vi "WM Spectra Stroke Calibration.vi"(0 "Input Time Series":dbl[](array[numeric]) format="%.2f", 1 "Water Depth":dbl format="%.2f", 2 "Sampling Rate":dbl format="%.2f", 3 "Paddle Height":dbl format="%.2f", 4 "Conversion Type":u16(ring) items=["Wave Height to Stroke", "Stroke to Wave Height"]) -> (5 "Output Time Series":dbl[](array[numeric]) format="%.2f")   [LabVIEW 2012]
uses:
  <vilib>/Analysis/2dsp.llb/Real FFT.vi
  <vilib>/Analysis/2dsp.llb/Inverse Real FFT.vi
  <vilib>/Analysis/NI_AALPro.lvlib
panel:
  # "Flap Stroke at Water line (S)"
  # "Flap Amplitude From x=0 (A')"
  # "Total Flap Stroke (S')"
  # "Flap Height (h')"
  # "Wave Height (Peak to trough) (H)"
  # "Wave Amplitude (z=0 to Peak) (A)"
  # "Wave Height to Flap Stroke at Water Line ( [H/S] )"
  # "Water Depth (h)"
  # "A' = h' * H / ( 2 * h * [H/S] )"
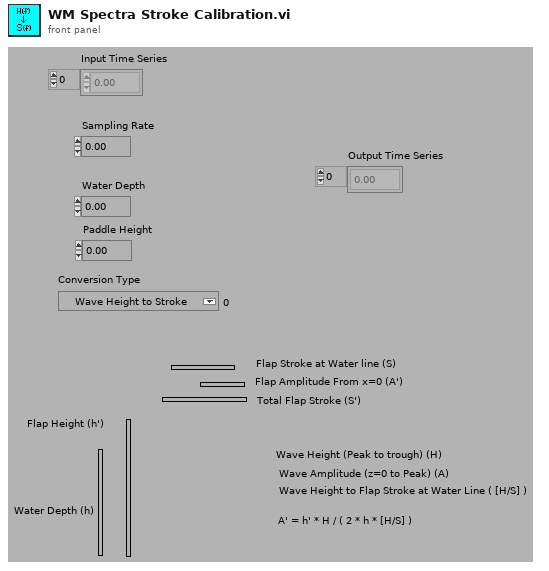
[diagram p1: front panel]
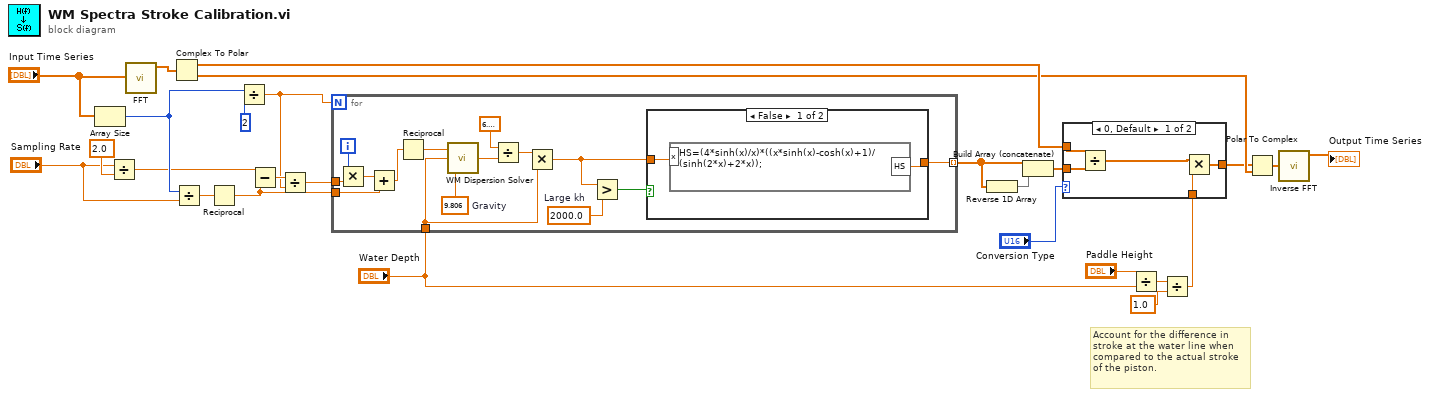
[diagram p0: block diagram]
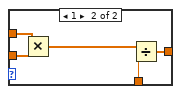
[diagram p2: hidden frame]
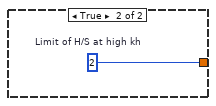
[diagram p3: hidden frame]
diagram:
  # "Account for the difference in \nstroke at the water line when \ncompared to the actual stroke\nof the piston."
  n1 = Array Size(array="Input Time Series") -> (size(s)=w14:i32)
  n2 = Divide(x="Sampling Rate", y=2.0) -> (x/y=w13:dbl)
  n3 = call-poly <vilib>:"FFT.vi"("X"="Input Time Series") -> ("FFT {X}"=w25:cdb[])  [unwired: 9 in, 1 out]
  n4 = Complex To Polar(r * e^(i*theta)=w25) -> (r=w24:dbl[], theta=w23:dbl[])
  n5 = Divide(x=w14, y="Sampling Rate") -> (x/y=w9:dbl)
  n6 = Reciprocal(x=w9) -> (1/x=w8:dbl)
  n7 = Divide(x=w14, y=2) -> (x/y=w11:dbl)
  n8 = Subtract(x=w13, y=w8) -> (x-y=w12:dbl)
  n9 = Divide(x=w12, y=w11) -> (x/y=w10:dbl)
  n10 = for {
    N: w11 -> [_]
    tunnel: w10 -> [w37]
    tunnel: "Water Depth" -> [w38]
    tunnel: w8 -> [w34]
    tunnel: [w31] -> w7 mode=indexing
    i -> [w36]
    w27 = 2000.0  # Large kh
    w30 = 9.806  # Gravity
    n11 = Multiply(x=w36, y=w37) -> (x*y=w35:dbl)
    n12 = Add(x=w35, y=w34) -> (x+y=w33:dbl)
    n13 = Reciprocal(x=w33) -> (1/x=w41:dbl)
    n14 = call "WM Dispersion Solver.vi"("Gravity"=w30, "Water Depth"=w38, "Wave Period"=w41) -> ("Wave Length"=w32:dbl)
    n15 = Divide(x=6.283185307179586, y=w32) -> (x/y=w39:dbl)
    n16 = Multiply(x=w39, y=w38) -> (x*y=w29:dbl)
    n17 = Greater?(x=w29, y=w27) -> (0:w28:bool)
    n18 = case shown="False" w28 {
      tunnel: [w42 w44] -> w31
      tunnel: w29 -> [w43 _]
      frame False {
        n19 = formula code="HS=(4*sinh(x)/x)*((x*sinh(x)-cosh(x)+1)/(sinh(2*x)+2*x));"("x"=w43) -> ("HS"=w42:dbl)
      }
      frame True {
        w44 = 2  # Limit of H/S at high kh
      }
    }
  }
  n20 = Reverse 1D Array(array=w7) -> (reversed array=w19:dbl[])
  n21 = Build Array (concatenate)(w7, w19) -> (w18:dbl[])
  n22 = Divide(x="Paddle Height", y="Water Depth") -> (x/y=w4:dbl)
  n23 = Divide(x=w4, y=1.0) -> (x/y=w2:dbl)
  n24 = case shown="0, Default" "Conversion Type" {
    tunnel: w24 -> [w49 w54]
    tunnel: w18 -> [w48 w53]
    tunnel: w2 -> [w46 w51]
    tunnel: [w45 w50] -> w1
    frame 0, Default {
      n25 = Divide(x=w49, y=w48) -> (x/y=w47:dbl[])
      n26 = Multiply(x=w47, y=w46) -> (x*y=w45:dbl[])
    }
    frame 1 {
      n27 = Multiply(x=w54, y=w53) -> (x*y=w52:dbl[])
      n28 = Divide(x=w52, y=w51) -> (x/y=w50:dbl[])
    }
  }
  n29 = Polar To Complex(1:w23, 2:w1) -> (0:w22:cdb[])
  n30 = call-poly <vilib>:"Inverse FFT.vi"("FFT {X}"=w22) -> ("X"=→"Output Time Series":dbl[])  [unwired: 9 in, 1 out]
